vi "Set Display Digits.vi"(8 "error in (no error)":errorcluster, 9 "Digit Values /Resolution":u16(ring) items=["3.5 digit resolution", "4.5 digit resolution", "5.5 digit resolution", "6.5 digit resolution", "7.5 digit resolution"], 10 "Function":u16(ring) items=["Voltage: DC", "Voltage: AC", "Current: DC", "Current: AC", "2W Resistance", "4W Resistance", "Diode", "Capacitance", "Temperature", "Continuity", "Frequency", "Period", "Ratio", "Digitize Voltage", "Digitize Current"], 11 "VISA resource name":refnum<visa-resource-name>) -> (0 "error out":errorcluster, 3 "VISA resource name out":refnum<visa-resource-name>)   [LabVIEW 2009, in "Keithley DMM7510.lvlib"]
doc: "This VI sets the number of digits that are displayed for measurements on the front panel."
uses:
  Keithley DMM7510.lvlib
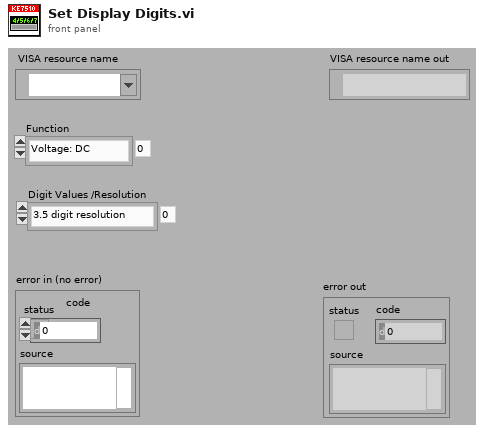
[diagram p1: front panel]
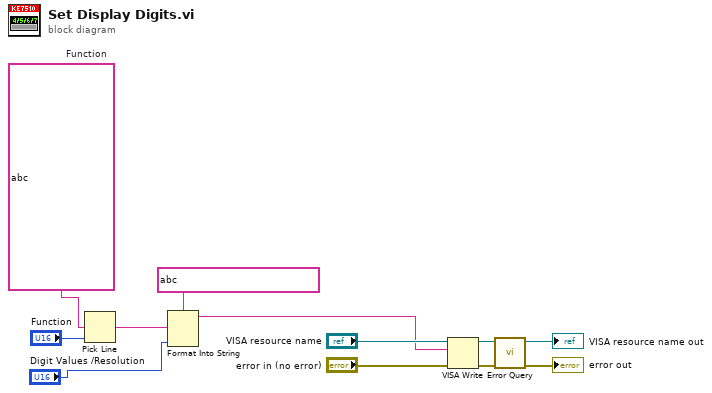
[diagram p0: block diagram]
diagram:
  w1 = string ?  # Function
  n1 = Pick Line(multi-line string=w1, line index="Function") -> (output string=w5:string)  [unwired: 1 in]
  n2 = Format Into String(format string=string ? ("write buffer"), w5, "Digit Values /Resolution") -> (resulting string=w4:string)  [unwired: 2 in, 1 out]
  n3 = VISA Write(VISA resource name="VISA resource name", write buffer=w4, error in (no error)="error in (no error)") -> (VISA resource name out=w8:refnum<visa-resource-name>, error out=w7:errorcluster)  [unwired: 1 out]
  n4 = call "Error Query.vi"("error in (no error)"=w7, "VISA resource name"=w8) -> ("error out"=→"error out":errorcluster, "VISA resource name out"=→"VISA resource name out":refnum<visa-resource-name>)  [unwired: 8 out]
